vi "AB_900_1000_Change_Path_from_Label.vi"(8 "error in (no error)":errorcluster, 9 "new label":string, 10 "old label":string, 11 "Path in":path) -> (0 "error out":errorcluster, 3 "Path out":path, 5 "changed?":bool)   [LabVIEW 2020]
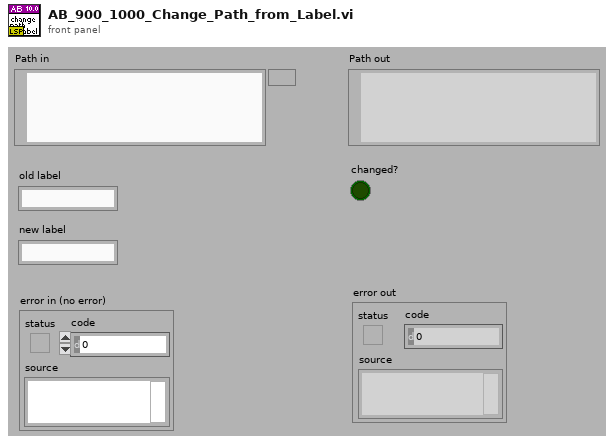
[diagram p1: front panel]
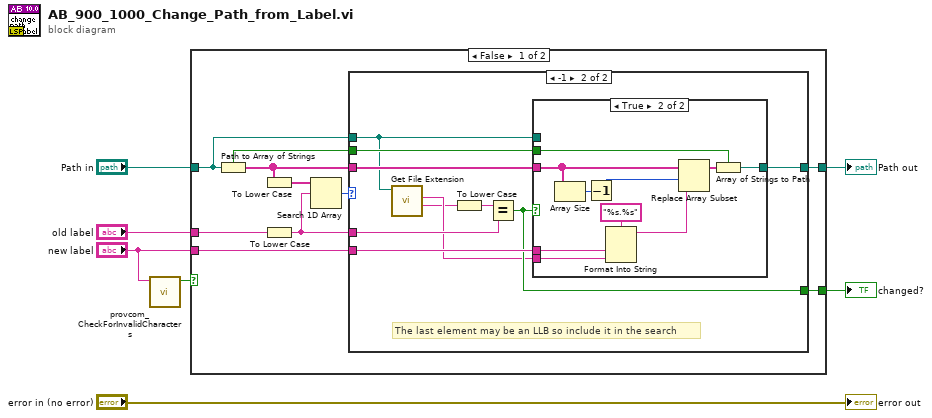
[diagram p0: block diagram]
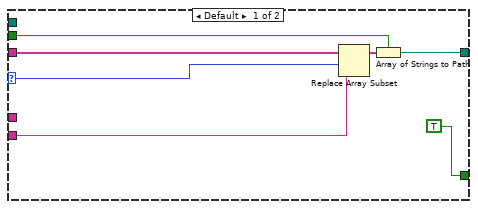
[diagram p2: hidden frame]
diagram:
  n1 = call <resource>:"provcom_CheckForInvalidCharacters.vi"("NewString"="new label") -> ("HasInvalidCharacters"=w1:bool)  [unwired: 9 in, 1 out]
  n2 = case shown="False" w1 {
    tunnel: [w16 w46] -> w7
    tunnel: "Path in" -> [w15 w46]
    tunnel: "old label" -> [w12 _]
    tunnel: [w9 _] -> w3
    tunnel: "new label" -> [w8 _]
    frame False {
      n3 = Path to Array of Strings(0:w15) -> (1:w17:bool, 2:w14:string[])
      n4 = To Lower Case(string=w14) -> (all lower case string=w13:string[])
      n5 = To Lower Case(string=w12) -> (all lower case string=w10:string)
      n6 = Search 1D Array(1D array=w13, element=w10) -> (index of element=w11:i32)  [unwired: 1 in]
      n7 = case shown="-1" w11 {
        selector: w11 -> [w20 _]
        tunnel: w17 -> [w23 w31]
        tunnel: w8 -> [w19 w30]
        tunnel: w14 -> [w22 w29]
        tunnel: [w21 w32] -> w16
        tunnel: w15 -> [_ w27]
        tunnel: w10 -> [_ w33]
        tunnel: [TRUE w28] -> w9
        frame Default {
          n8 = Replace Array Subset(array=w22, new element=w19, index=w20) -> (w24:string[])
          n9 = Array of Strings to Path(0:w24, 1:w23) -> (2:w21:path)
        }
        frame -1 {
          # "The last element may be an LLB so include it in the search"
          n10 = call <vilib>:"Get File Extension.vi"("file"=w27) -> ("filename without extension"=w25:string, "lowercase file extension"=w26:string)  [unwired: 6 in, 3 out]
          n11 = To Lower Case(string=w25) -> (all lower case string=w34:string)
          n12 = Equal?(x=w34, y=w33) -> (x = y?=w28:bool)
          n13 = case shown="True" w28 {
            tunnel: [w35 w44] -> w32
            tunnel: w31 -> [_ w43]
            tunnel: w26 -> [_ w36]
            tunnel: w30 -> [_ w38]
            tunnel: w29 -> [_ w42]
            tunnel: w27 -> [w35 _]
            frame False {
            }
            frame True {
              n14 = Array Size(array=w42) -> (size(s)=w41:i32)
              n15 = Decrement(x=w41) -> (x-1=w40:i32)
              n16 = Format Into String(format string="%s.%s", w38, w36) -> (resulting string=w37:string)  [unwired: 2 in, 1 out]
              n17 = Replace Array Subset(array=w42, new element=w37, index=w40) -> (w45:string[])
              n18 = Array of Strings to Path(0:w45, 1:w43) -> (2:w44:path)
            }
          }
        }
      }
    }
    frame True {
      # "The label is just a string so it can have invalid path characters. If it does, don't change the path."
    }
  }
  "Path out" <- w7
  "changed?" <- w3
  "error out" <- "error in (no error)"
